vi "Waveform-Create (contin).vi"(8 "error in (no error)":errorcluster, 9 "sampling info":T18={"Fs"=1000.0, "N"=1000} {"Fs" format="%.2p"}, 10 "Old Waveform":T17(xcontrol), 11 "New Waveform":T17(xcontrol)) -> (0 "error out":errorcluster, 2 "Signal":dbl[](array[numeric]), 3 "Waveform Out":T17(xcontrol))   [LabVIEW 2015]
doc: "Takes a generic waveform description and returns a token of the specific waveform."
uses:
  Controls/Waveform XCtl/Waveform XCtl.xctl
  Controls/Typedefs/Sampling Info.ctl
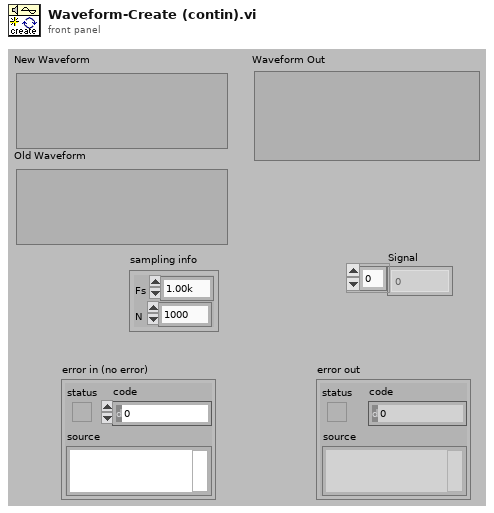
[diagram p1: front panel]
types:
  T1 = typedef "Waveform Enum.ctl" = enum16{"OFF", "Tone", "Noise", "Pulse Train", "File", "FM Sweep", "Chirp Train", "Complex Tone", "FM Tone", "Moving Ripple"}
  T2 = typedef "Tone Params.ctl" = cluster{"Frequency (kHz)":dbl, "Last Freq":dbl, "Last Phase":dbl}
  T3 = typedef "Pulse Train Params.ctl" = cluster{"Pulse width (us)":dbl, "Pulse rate (Hz)":dbl, "Gap (ms)":dbl, "Polarity":T4, "PT State":T5, "Asynch":bool}
  T4 = typedef "Pulse Polarity.ctl" = enum16{"POS", "NEG", "POS-NEG", "NEG-POS"}
  T5 = typedef "PT-Continuous State.ctl" = cluster{"Template":dbl[], "Nperiod":i32, "Index":i32, "Pulse Rate (Hz)":dbl, "Phase (cycles)":dbl, "Noff":i32}
  T6 = typedef "Noise Params.ctl" = cluster{"InvFilt":bool, "Noise":dbl[], "CurPt":i32, "Aweight":bool, "Seed":i32, "afile":path}
  T7 = typedef "StimFile-Params.ctl" = cluster{"Filename":path, "Signal":dbl[], "Channel":i32, "stream":bool, "offset":i32, "nreps":i32, "loops":i32, "Tokens":i32, "Randomize":bool, "order":i32[]}
  T8 = typedef "FM Sweep Params.ctl" = cluster{"Rate (oct/s)":dbl, "Fmin (Hz)":dbl, "Fmax (Hz)":dbl, "Ramp (ms)":dbl, "Linear":bool}
  T9 = typedef "Chirp Train.ctl" = cluster{"Params":T10, "Data":cluster{"WF":dbl[]}}
  T10 = typedef "Chirp Train Params.ctl" = cluster{"Fmin (kHz)":dbl, "Fmax (kHz)":dbl, "Compensate":bool, "Duration (ms)":dbl}
  T11 = typedef "CT-Params.ctl" = cluster{"F0 (Hz)":dbl, "Band":cluster{"Flow (Hz)":dbl, "Fhigh (Hz)":dbl}, "Phase":T12, "Min F0 (Hz)":dbl, "Max F0 (Hz)":dbl, "ContinRandPhase":bool, "Max peak factor":dbl, "Max mod depth":dbl, "MinHarmNum":i32, "MaxHarmNum":i32, "Level Mode":enum16{"per component", "overall rms"}, "% jitter":dbl}
  T12 = typedef "CT-Phase Enum.ctl" = enum16{"Cosine", "Random", "Alternating"}
  T13 = typedef "CT-Runtime Data.ctl" = cluster{"Ncomp":i32, "MinHarm":i32, "Phase":dbl[], "Amplitude":dbl[], "Npts/frame":i32, "Last F0":dbl, "Fmin":dbl, "Fmax":dbl, "Lslope":dbl, "randphase":bool, "overall rms":bool, "fmult":dbl[], "jittered":bool}
  T14 = typedef "Moving Ripple.ctl" = cluster{"Params":T15, "Data":T16}
  T15 = typedef "Moving Ripple.Params.ctl" = cluster{"Fmin":dbl, "Fmax":dbl, "Density":dbl, "Velocity":dbl, "Depth":dbl, "Phase":dbl, "Comp/oct":i32}
  T16 = typedef "Moving Ripple.Data.ctl" = cluster{"Freq":dbl[], "A":dbl[], "phase":dbl[], "Phase":dbl}
  T17 = cluster{"Type":T1, "Tone":T2, "Pulse Train":T3, "Noise":T6, "File":T7, "FMSweep":T8, "Chirp Train":T9, "Complex Tone":cluster{"Params":T11, "Data":T13}, "Moving Ripple":T14}
  T18 = typedef "Sampling Info.ctl" = cluster{"Fs":dbl, "N":i32}
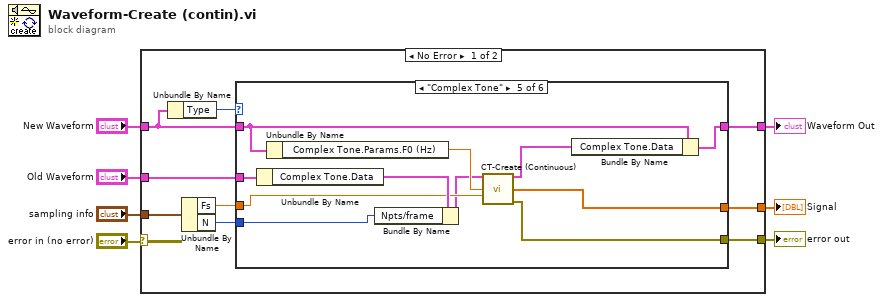
[diagram p0: block diagram]
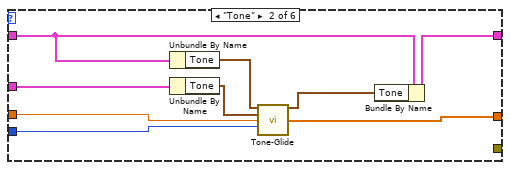
[diagram p3: hidden frame]
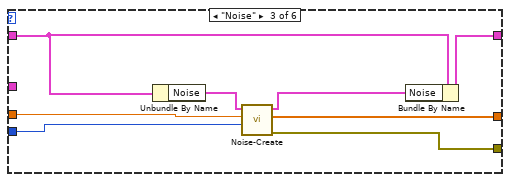
[diagram p4: hidden frame]
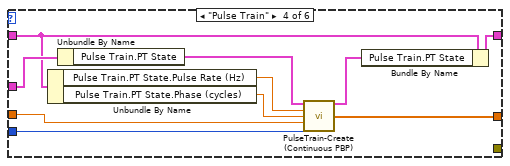
[diagram p5: hidden frame]
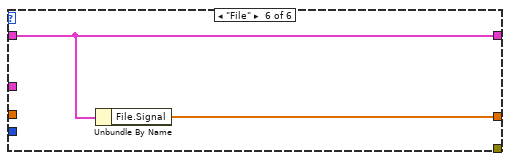
[diagram p6: hidden frame]
diagram:
  n1 = case shown="No Error" "error in (no error)" {
    selector: "error in (no error)" -> [_ w59]
    tunnel: [w15 w59] -> w6
    tunnel: "New Waveform" -> [w8 w58]
    tunnel: [w14 _] -> w5
    tunnel: [w13 w58] -> w4
    tunnel: "sampling info" -> [w11 _]
    tunnel: "Old Waveform" -> [w9 _]
    frame No Error {
      n2 = Unbundle By Name(w8) -> ("Type"=w16:T1)
      n3 = Unbundle By Name(w11) -> ("Fs"=w12:dbl, "N"=w10:i32)
      n4 = case shown="\"Complex Tone\"" w16 {
        tunnel: w12 -> [_ w21 w34 w43 w52 _]
        tunnel: w10 -> [_ w26 w33 w42 w50 _]
        tunnel: w8 -> [w17 w25 w31 w35 w47 w57]
        tunnel: [_ _ w29 _ w48 _] -> w15
        tunnel: [_ w20 w28 w44 w49 w56] -> w14
        tunnel: [w17 w24 w27 w40 w45 w57] -> w13
        tunnel: w9 -> [_ w19 _ w36 w55 _]
        frame "OFF", Default {
        }
        frame "Tone" {
          n5 = Unbundle By Name(w25) -> ("Tone"=w23:T2)
          n6 = Unbundle By Name(w19) -> ("Tone"=w18:T2)
          n7 = call "Tone-Glide.vi"("New"=w23, "Old"=w18, "Fs (Hz)"=w21, "Npts"=w26) -> ("Params out"=w22:T2, "Y"=w20:dbl[])  [unwired: 10 in]
          n8 = Bundle By Name(cluster=w25, "Tone"=w22) -> (w24:T17)
        }
        frame "Noise" {
          n9 = Unbundle By Name(w31) -> ("Noise"=w32:T6)
          n10 = call "Noise-Create.vi"("Npts"=w33, "Sampling Rate (Hz)"=w34, "Noise Params"=w32) -> ("error out"=w29:errorcluster, "Waveform"=w28:dbl[], "Noise Params (out)"=w30:T6)  [unwired: 6 in]
          n11 = Bundle By Name(cluster=w31, "Noise"=w30) -> (w27:T17)
        }
        frame "Pulse Train" {
          n12 = Unbundle By Name(w35) -> ("Pulse Train.PT State.Pulse Rate (Hz)"=w38:dbl, "Pulse Train.PT State.Phase (cycles)"=w37:dbl)
          n13 = Unbundle By Name(w36) -> ("Pulse Train.PT State"=w41:T5)
          n14 = call "PulseTrain-Create (Continuous PBP).vi"("State In"=w41, "Pulse Rate (Hz)"=w38, "Phase (cycles)"=w37, "Fs (Hz)"=w43, "Npts"=w42) -> ("State Out"=w39:T5, "Buffer"=w44:dbl[])  [unwired: 8 in, 1 out]
          n15 = Bundle By Name(cluster=w35, "Pulse Train.PT State"=w39) -> (w40:T17)
        }
        frame "Complex Tone" {
          n16 = Unbundle By Name(w55) -> ("Complex Tone.Data"=w54:T13)
          n17 = Unbundle By Name(w47) -> ("Complex Tone.Params.F0 (Hz)"=w53:dbl)
          n18 = Bundle By Name(cluster=w54, "Npts/frame"=w50) -> (w51:T13)
          n19 = call "CT-Create (Continuous).vi"("HCT Runtime in"=w51, "F0 (Hz)"=w53, "Fs (Hz)"=w52) -> ("HCT Runtime out"=w46:T13, "HCT"=w49:dbl[], "error out"=w48:errorcluster)  [unwired: 10 in]
          n20 = Bundle By Name(cluster=w47, "Complex Tone.Data"=w46) -> (w45:T17)
        }
        frame "File" {
          n21 = Unbundle By Name(w57) -> ("File.Signal"=w56:dbl[])
        }
      }
    }
    frame Error {
    }
  }
  "error out" <- w6
  "Signal" <- w5
  "Waveform Out" <- w4
